vi "AccelTankDrive.vi"(8 "Right":dbl, 11 "Left":dbl) -> ()   [LabVIEW 2015]
uses:
  <vilib>/Rock Robotics/WPI/Utilities/WPI_GetSetVariantRefNum.vi
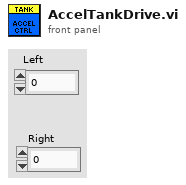
[diagram p1: front panel]
types:
  T1 = typedef "WPI_RobotDriveDevRef.ctl" = cluster{"DevStatus":errorcluster, "Motors[]":T2[], "Square Inputs":bool, "Max Output":dbl}
  T2 = typedef "WPI_MotorControlDeviceRef.ctl" = cluster{"DeviceStatus":errorcluster, "Type":T3, "PWM":cluster{"PWM Channel":T4, "DeadBand":T5}, "CAN":cluster{"Device Number":u8, "Control Mode":T6, "Semaphore":T7, "Max Vout":dbl, "TalonSRX Control Mode":T8}, "Invert":bool}
  T3 = typedef "WPI_MotorControlType.ctl" = enum16{"PWM", "CAN", "CANTalonSRX"}
  T4 = typedef "FPGA_DIOPWMChannel.ctl" = enum8{"PWM 0", "PWM 1", "PWM 2", "PWM 3", "PWM 4", "PWM 5", "PWM 6", "PWM 7", "PWM 8", "PWM 9", "PWM MXP 0", "PWM MXP 1", "PWM MXP 2", "PWM MXP 3", "PWM MXP 4", "PWM MXP 5", "PWM MXP 6", "PWM MXP 7", "PWM MXP 8", "PWM MXP 9", "Invalid"}
  T5 = typedef "WPI_PWMDeadband.ctl" = cluster{"Name":string, "maxPositivePwm":i32, "minPositivePwm":i32, "centerPwm":i32, "maxNegativePwm":i32, "minNegativePwm":i32, "angularRange":u16}
  T6 = typedef "WPI_CANJaguar_ControlMode.ctl" = enum8{"Percent VBus", "Current", "Speed", "Position", "Voltage"}
  T7 = typedef "Semaphore RefNum" = refnum<k1>
  T8 = typedef "WPI_CANTalonSRX_APIControlMode.ctl" = enum8{"Percent VBus", "Speed", "Position", "Slave", "Unchanged / Invalid", "Voltage Compensation", "Current", "Motion Profile"}
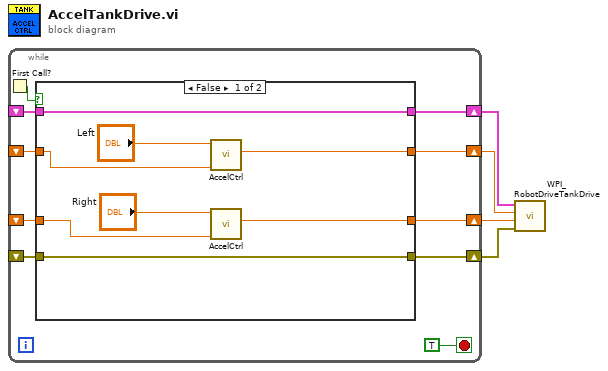
[diagram p0: block diagram]
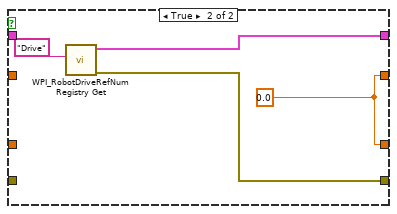
[diagram p2: hidden frame]
diagram:
  n1 = while {
    shift-right: [w13] -> w4
    shift-left: _ -> [w9]
    shift-right: [w12] -> w3
    shift-left: _ -> [w8]
    shift-right: [w10] -> w1
    shift-left: _ -> [w7]
    shift-right: [w11] -> w2
    shift-left: _ -> [w6]
    stop <- TRUE stop-if-true
    n2 = First Call?() -> (First Call?: T/F=w14:bool)
    n3 = case shown="False" w14 {
      tunnel: [w22 w25] -> w13
      tunnel: [w21 w24] -> w12
      tunnel: [w19 w23] -> w11
      tunnel: [w20 w23] -> w10
      tunnel: w9 -> [w22 _]
      tunnel: w8 -> [w21 _]
      tunnel: w7 -> [w16 _]
      tunnel: w6 -> [w15 _]
      frame False {
        n4 = call "AccelCtrl.vi"("CurrentSpeed"=w16, "TargetSpeed"="Left") -> ("Speed"=w20:dbl)  [unwired: 9 in]
        n5 = call "AccelCtrl.vi"("CurrentSpeed"=w15, "TargetSpeed"="Right") -> ("Speed"=w19:dbl)  [unwired: 9 in]
      }
      frame True {
        w23 = 0.0
        n6 = call <vilib>:"WPI_RobotDriveRefNum Registry Get.vi"("refnum name"="Drive") -> ("error out"=w24:errorcluster, "RobotDriveDevRef"=w25:T1)  [unwired: 9 in]
      }
    }
  }
  n7 = call <vilib>:"WPI_RobotDriveTankDrive.vi"("error in (no error)"=w3, "Right axis value"=w2, "Left axis value"=w1, "RobotDriveDevRef"=w4) -> ()  [unwired: 5 in, 3 out]
